vi "CCSA RPJ SLJC PR002 SubVI002.vi"(1 "Derecha":T1, 2 "Izquierda":T1) -> (0 "Array":u16[][](array[numeric]))   [LabVIEW 2021]
doc: "Realiza la segmentación de la imagen y porterior a ello obtiene los centroides, tres por cada imagen para objetos Rojo, verde y azul. Recibe un arreglo de dos imágenes y regresa una matriz de [2x3]."
uses:
  <vilib>/vision/Image Controls.llb/IMAQ Image.ctl
panel:
  # "CUEVAS CERÓN SERGIO ALBERTO\nREYES PÉREZ JAVIER\nSALCEDO LICEA JUAN CARLOS"
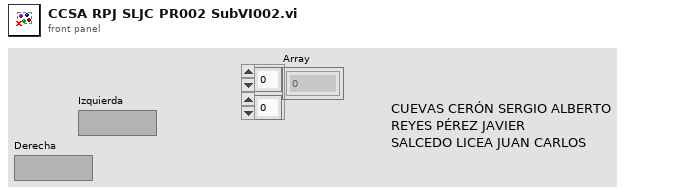
[diagram p1: front panel]
types:
  T1 = typedef "IMAQ Image.ctl" = refnum<image>
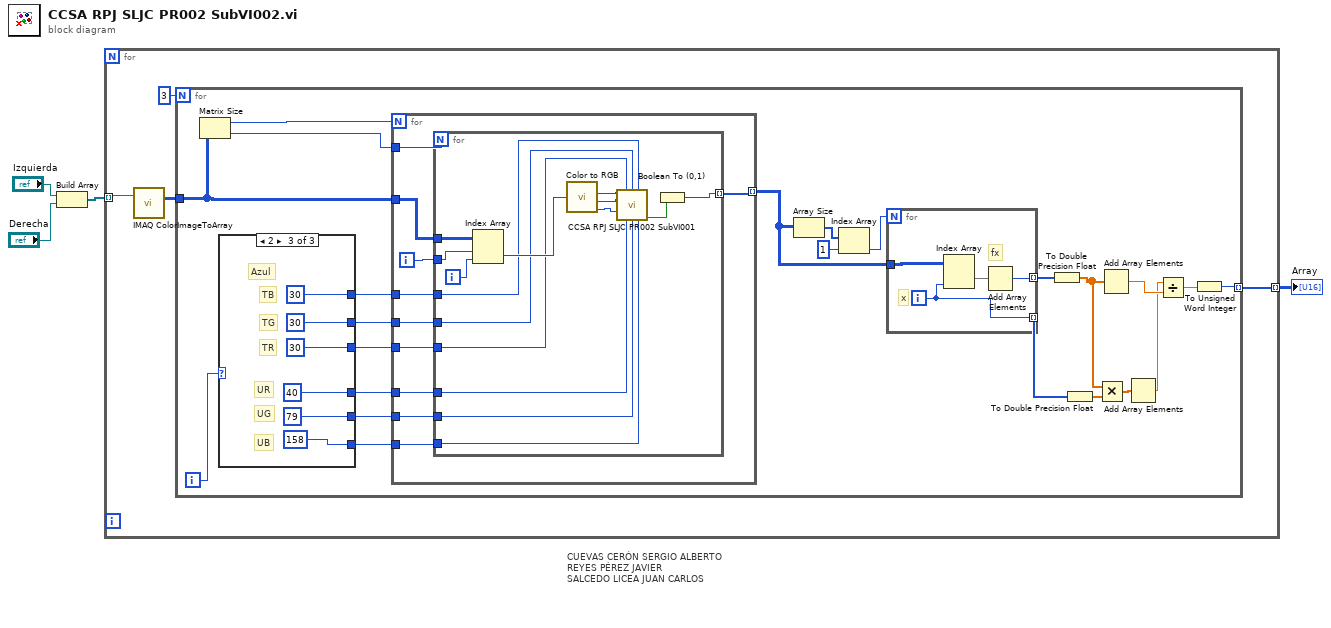
[diagram p0: block diagram]
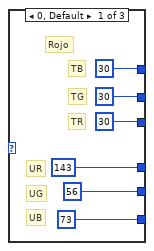
[diagram p2: hidden frame]
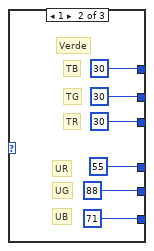
[diagram p3: hidden frame]
diagram:
  # "CUEVAS CERÓN SERGIO ALBERTO\nREYES PÉREZ JAVIER\nSALCEDO LICEA JUAN CARLOS"
  n1 = Build Array("Izquierda", "Derecha") -> (w2:T1[])
  n2 = for {
    tunnel: [w7] -> w1 mode=indexing
    tunnel: w2 -> [w5] mode=indexing
    n3 = call "IMAQ ColorImageToArray"("Image"=w5) -> ("Image Pixels (U32)"=w6:u32[][])  [unwired: 3 in, 2 out]
    n4 = for {
      N: 3 -> [_]
      tunnel: w6 -> [w31]
      tunnel: [w22] -> w7 mode=indexing
      i -> [w21]
      n5 = Matrix Size(0:w31) -> (1:w30:i32, 2:w29:i32)
      n6 = case shown="2" w21 {
        tunnel: [u8 143 ("umbralVerde") u8 55 ("umbralVerde") u8 40 ("umbralVerde")] -> w20
        tunnel: [u8 56 ("umbralRojo") u8 88 ("umbralRojo") u8 79 ("umbralRojo")] -> w19
        tunnel: [u8 73 ("umbralAzul") u8 71 ("umbralAzul") u8 158 ("umbralAzul")] -> w18
        tunnel: [u8 30 ("tolerancia") u8 30 ("tolerancia") u8 30 ("tolerancia")] -> w11
        tunnel: [u8 30 ("tolerancia") u8 30 ("tolerancia") u8 30 ("tolerancia")] -> w10
        tunnel: [u8 30 ("tolerancia") u8 30 ("tolerancia") u8 30 ("tolerancia")] -> w9
        frame 0, Default {
          # "Rojo"
          # "TR"
          # "TG"
          # "TB"
          # "UB"
          # "UG"
          # "UR"
        }
        frame 1 {
          # "Verde"
          # "TR"
          # "TG"
          # "TB"
          # "UB"
          # "UG"
          # "UR"
        }
        frame 2 {
          # "Azul"
          # "TR"
          # "TG"
          # "TB"
          # "UB"
          # "UG"
          # "UR"
        }
      }
      n7 = for {
        N: w30 -> [_]
        tunnel: w31 -> [w59]
        tunnel: w29 -> [w57]
        tunnel: [w56] -> w25 mode=indexing
        tunnel: w20 -> [w55]
        tunnel: w19 -> [w54]
        tunnel: w18 -> [w53]
        tunnel: w11 -> [w52]
        tunnel: w10 -> [w51]
        tunnel: w9 -> [w50]
        i -> [w58]
        n8 = for {
          N: w57 -> [_]
          tunnel: w59 -> [w73]
          tunnel: w58 -> [w72]
          tunnel: [w60] -> w56 mode=indexing
          tunnel: w55 -> [w65]
          tunnel: w54 -> [w66]
          tunnel: w53 -> [w67]
          tunnel: w52 -> [w63]
          tunnel: w51 -> [w62]
          tunnel: w50 -> [w61]
          i -> [w71]
          n9 = Index Array(array=w73, index (row)=w72, index (col)=w71) -> (element=w74:u32)
          n10 = call <vilib>:"Color to RGB.vi"("Color"=w74) -> ("R"=w70:u8, "G"=w69:u8, "B"=w68:u8)  [unwired: 1 out]
          n11 = call "CCSA RPJ SLJC PR002 SubVI001.vi"("R"=w70, "TR"=w61, "TG"=w62, "TB"=w63, "G"=w69, "B"=w68, "UR"=w65, "UG"=w66, "UB"=w67) -> ("binario"=w64:bool)  [unwired: 5 in, 1 out]
          n12 = Boolean To (0,1)(Boolean=w64) -> (0, 1=w60:i16)
        }
      }
      n13 = Array Size(array=w25) -> (size(s)=w28:i32[])
      n14 = Index Array(array=w28, index=1) -> (element=w26:i32)
      n15 = for {
        N: w26 -> [_]
        tunnel: w25 -> [w78]
        tunnel: [w76] -> w15 mode=indexing
        tunnel: [w75] -> w17 mode=indexing
        i -> [w75]
        # "x"
        # "fx"
        n16 = Index Array(array=w78, index (col)=w75) -> (element=w77:i16[])  [unwired: 1 in]
        n17 = Add Array Elements(numeric array=w77) -> (sum=w76:i16)
      }
      n18 = To Double Precision Float(number=w15) -> (double precision float=w12:dbl[])
      n19 = To Double Precision Float(number=w17) -> (double precision float=w16:dbl[])
      n20 = Multiply(x=w12, y=w16) -> (x*y=w24:dbl[])
      n21 = Add Array Elements(numeric array=w12) -> (sum=w14:dbl)
      n22 = Add Array Elements(numeric array=w24) -> (sum=w13:dbl)
      n23 = Divide(x=w13, y=w14) -> (x/y=w23:dbl)
      n24 = To Unsigned Word Integer(number=w23) -> (unsigned 16bit integer=w22:u16)
    }
  }
  "Array" <- w1
